vi "Sonar.vi"() -> (3 "distance":dbl(slide)=125.0 scale=0.0..250.0 scale format="%3d")   [LabVIEW 2013]
panel:
  in  "Scaling factor (V/in)":dbl=0.0098
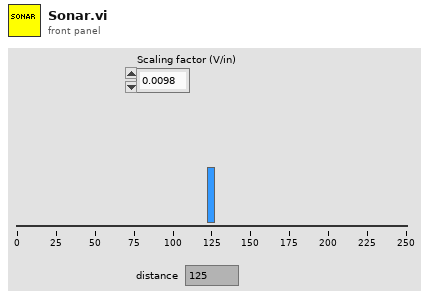
[diagram p1: front panel]
types:
  T1 = typedef "WPI_AnalogChannelDevRef.ctl" = cluster{"DevStatus":errorcluster, "Analog Module":T2, "Analog Channel":T3}
  T2 = typedef "FPGA_TypedefAnalogModule.ctl" = enum16{"Analog Module 1", "Analog Module 2"}
  T3 = typedef "FPGA_AIChannel.ctl" = enum8{"AI 1", "AI 2", "AI 3", "AI 4", "AI 5", "AI 6", "AI 7", "AI 8", "Invalid"}
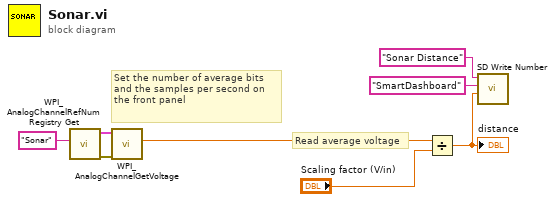
[diagram p0: block diagram]
diagram:
  # "Read average voltage"
  # "Set the number of average bits and the samples per second on the front panel"
  n1 = call <vilib>:"WPI_AnalogChannelRefNum Registry Get.vi"("refnum name"="Sonar") -> ("error out"=w2:errorcluster, "AIDeviceRef"=w3:T1)  [unwired: 9 in]
  n2 = call <vilib>:"WPI_AnalogChannelGetVoltage.vi"("error in (no error)"=w2, "AIDeviceRef"=w3) -> ("Voltage"=w1:dbl)  [unwired: 7 in, 2 out]
  n3 = Divide(x=w1, y="Scaling factor (V/in)") -> (x/y=w5:dbl)
  "distance" <- w5
  n4 = call <vilib>:"SD Write Number.vi"("Numeric"=w5, "Table Prefix"="SmartDashboard", "Name"="Sonar Distance") -> ()  [unwired: 7 in, 2 out]
